vi "Get Level Helium.vi"(8 "error in (no error)":errorcluster, 11 "instrument.PPMS2 in":refnum<class "instrument.PPMS2.lvclass">) -> (0 "error out":errorcluster, 2 "LHe Level (%)":dbl, 3 "instrument.PPMS2 out":refnum<class "instrument.PPMS2.lvclass">)   [LabVIEW 2016, in "instrument.PPMS2.lvclass"]
uses:
  instrument.PPMS2.lvclass
panel:
  in  "Data":variant
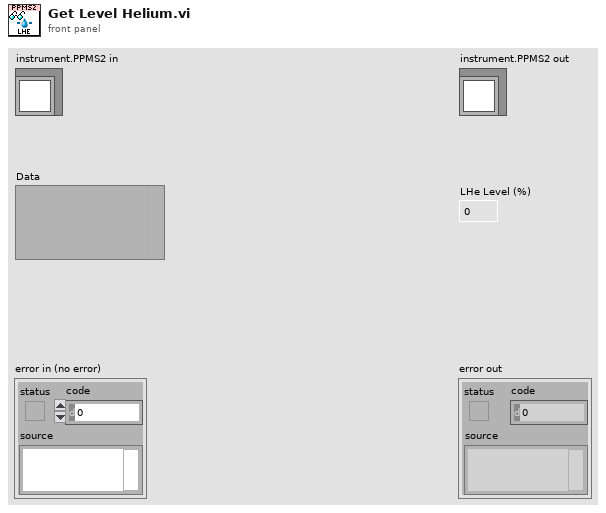
[diagram p1: front panel]
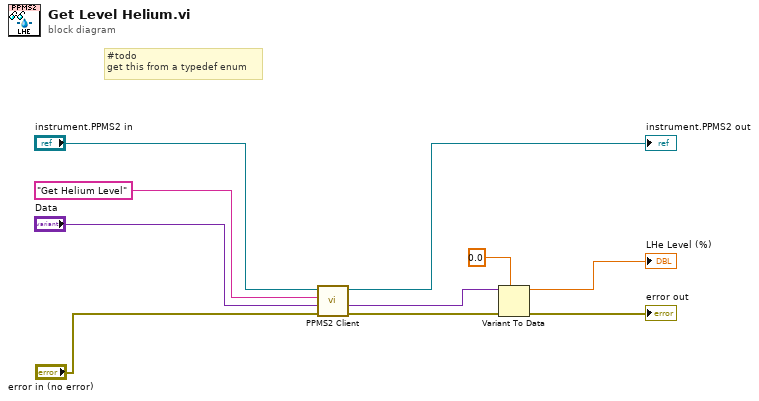
[diagram p0: block diagram]
diagram:
  # "#todo\nget this from a typedef enum"
  n1 = call "PPMS2 Client.vi"("error in (no error)"="error in (no error)", "Data"="Data", "Command"="Get Helium Level", "instrument.PPMS2 in"="instrument.PPMS2 in") -> ("error out"=w8:errorcluster, "Data out"=w3:variant, "instrument.PPMS2 out"=→"instrument.PPMS2 out":refnum<class "instrument.PPMS2.lvclass">)  [unwired: 4 in, 1 out]
  n2 = Variant To Data(error in=w8, type=0.0, Variant=w3) -> (data=→"LHe Level (%)":dbl, error out=→"error out":errorcluster)
